vi "Close and Unregister Events.vi"(8 "error in (no error)":errorcluster, 10 "user event in":refnum<user-event>, 11 "Event Registration Refnum in":refnum<event-registration>) -> (0 "error out":errorcluster)   [LabVIEW 2019]
uses:
  Controls/Commands.ctl
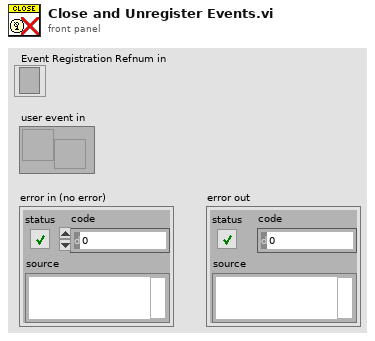
[diagram p1: front panel]
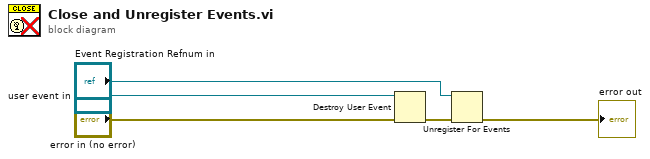
[diagram p0: block diagram]
diagram:
  n1 = Destroy User Event(user event="user event in", error in="error in (no error)") -> (error out=w3:errorcluster)
  n2 = Unregister For Events(event registration refnum="Event Registration Refnum in", error in=w3) -> (error out=→"error out":errorcluster)
